vi "TL forebrain THINK.vi"(7 "MDF":T1(array[cluster]), 8 "error in":errorcluster, 9 "Run?":bool=TRUE, 10 "MDF index":i32, 11 "GPS":cluster{"X pos":i32, "Y pos":i32, "Heading":dbl}={"X pos"=250, "Y pos"=250, "Heading"=0.0}) -> (0 "error out":errorcluster, 1 "local Steering\nangle":dbl, 2 "MDF Index out":i32, 3 "Behaviors out":T2, 5 "MDF Out":T1(array[cluster]), 6 "Complete?":bool=TRUE)   [LabVIEW 2014]
panel:
  out "At Waypoint?":bool
  out "Forebrain Command":T3
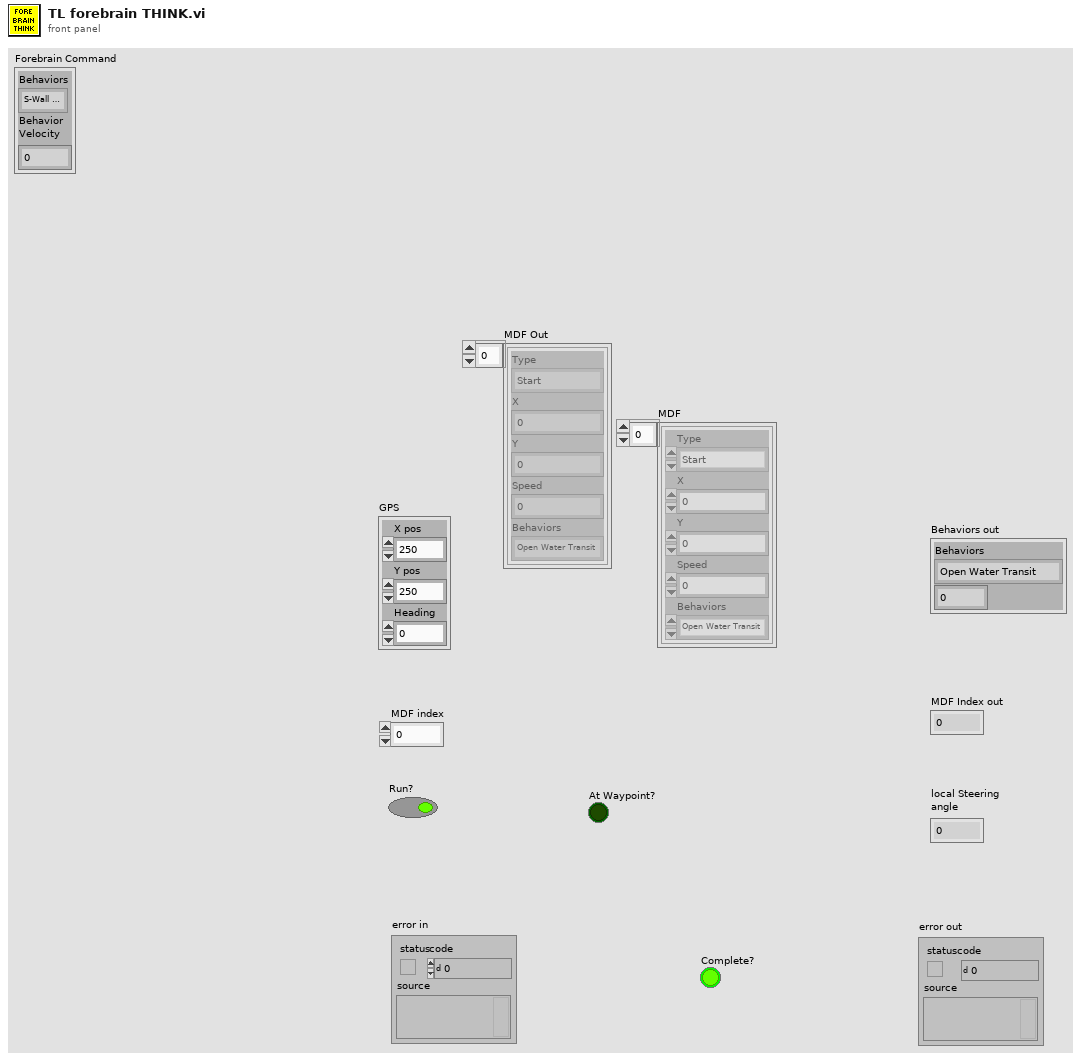
[diagram p1: front panel]
types:
  T1 = cluster{"Type":enum16{"Start", "Buoy Circling", "Waypoint", "End"}, "X":i32, "Y":i32, "Speed":i32, "Behaviors":enum16{"Open Water Transit", "P-Wall Follow", "S-Wall Follow", "Get Unstuck"}}[]
  T2 = cluster{"Behaviors":enum16{"Open Water Transit", "P-Wall Follow", "S-Wall Follow", "Get Unstuck"}, dbl}
  T3 = cluster{"Behaviors":enum16{"S-Wall Follow", "P-Wall Follow", "Open Water Transit", "Get Unstuck"}, "Behavior\nVelocity":dbl}
  T4 = enum16{"Open Water Transit", "P-Wall Follow", "S-Wall Follow", "Get Unstuck"}
  T5 = cluster{"Type":enum16{"Start", "Buoy Circling", "Waypoint", "End"}, "X":i32, "Y":i32, "Speed":i32, "Behaviors":enum16{"Open Water Transit", "P-Wall Follow", "S-Wall Follow", "Get Unstuck"}}
  T6 = enum16{"Start", "Buoy Circling", "Waypoint", "End"}
  T7 = cluster{"Pos. X":i32, "Pos. Y":i32, "Radius":i32, "Core Area":i32}[]
  T8 = cluster{"Pos. X":i32, "Pos. Y":i32, "Radius":i32, "Core Area":i32}
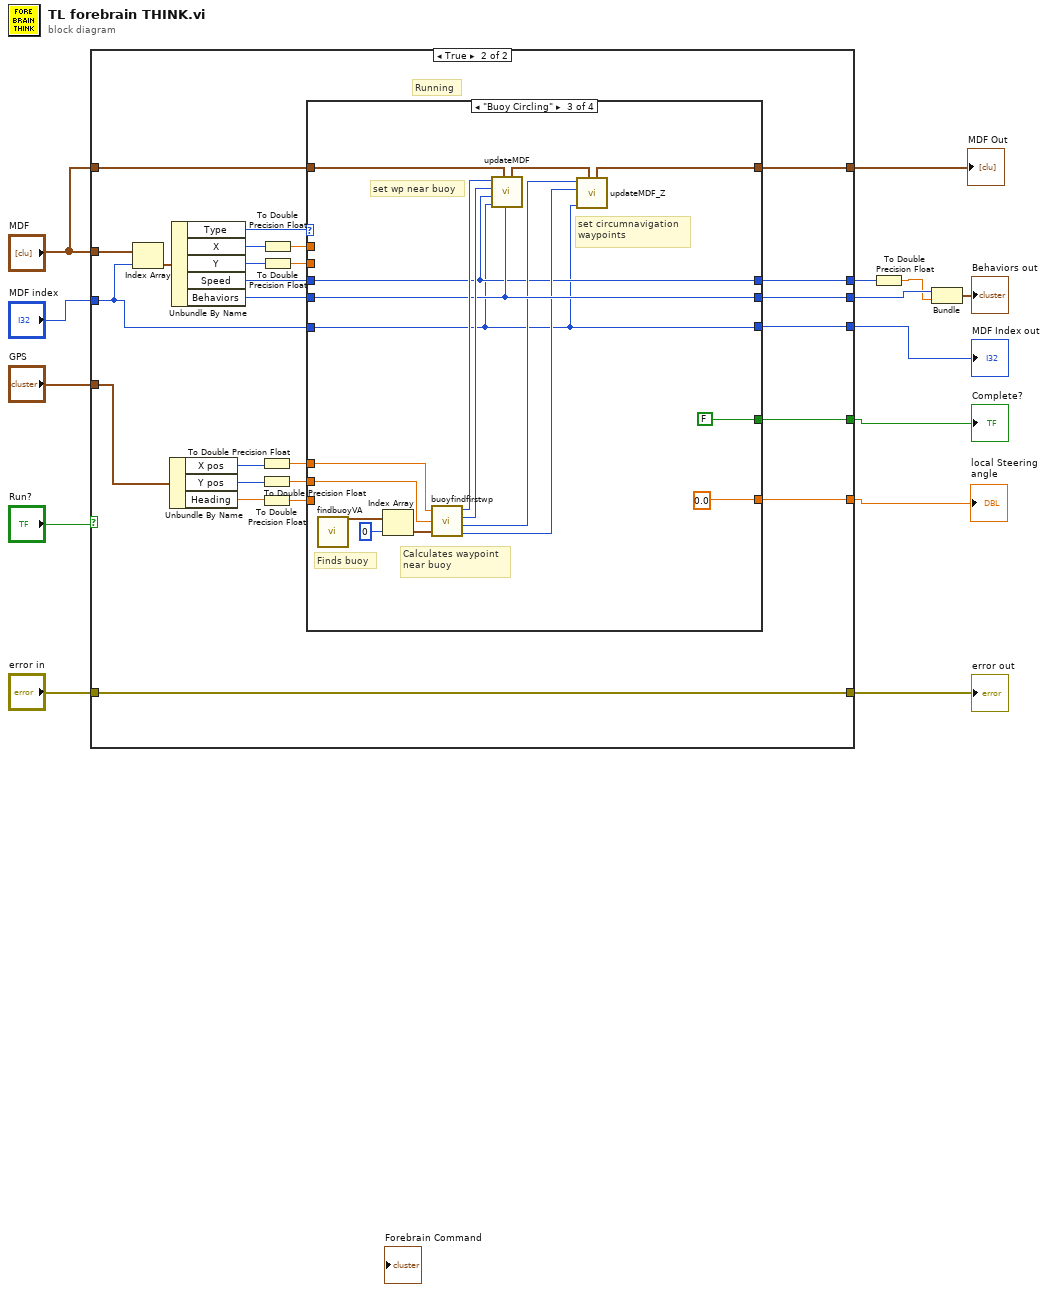
[diagram p0: block diagram]
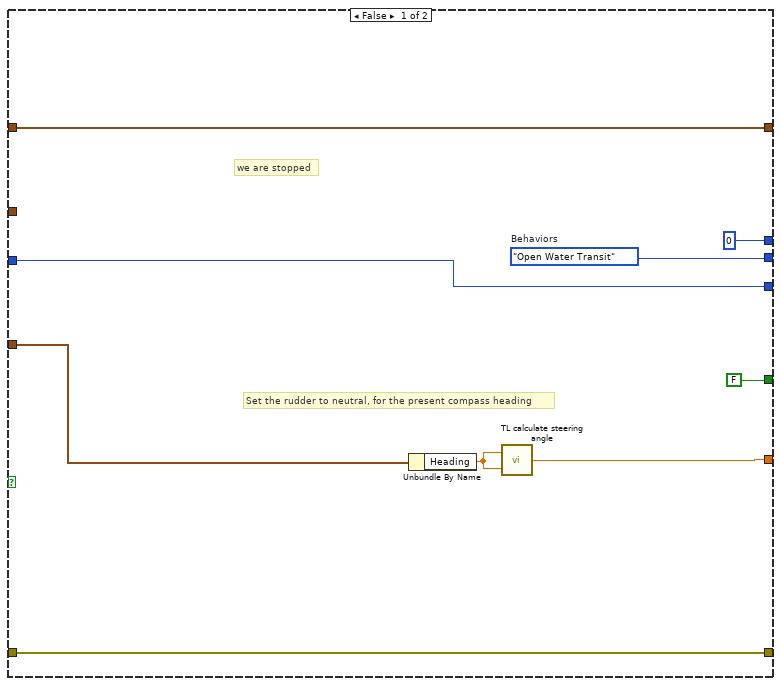
[diagram p2: hidden frame]
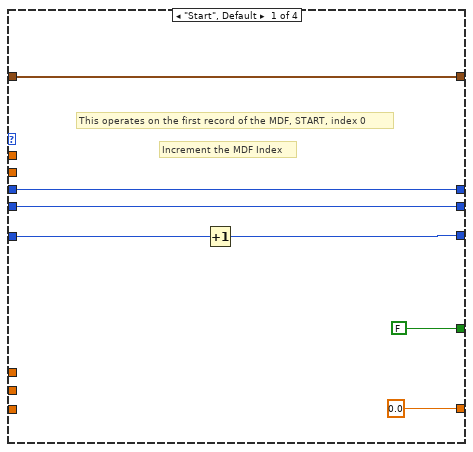
[diagram p3: hidden frame]
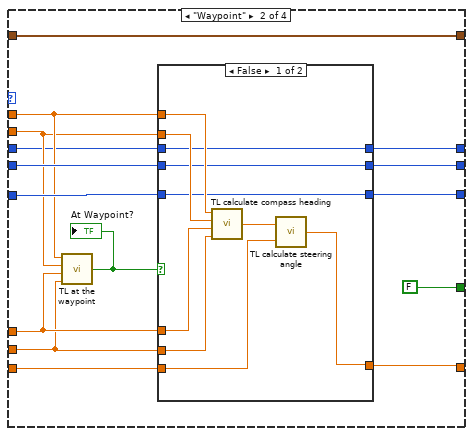
[diagram p4: hidden frame]
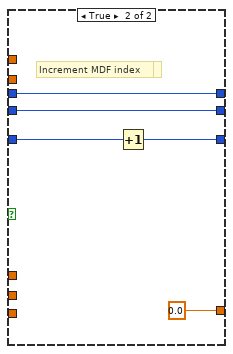
[diagram p5: hidden frame]
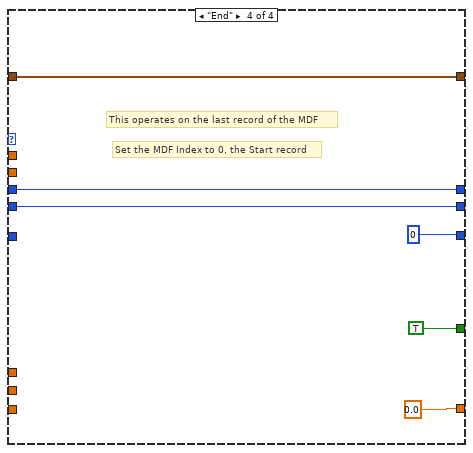
[diagram p6: hidden frame]
diagram:
  n1 = case shown="True" "Run?" {
    tunnel: "MDF" -> [_ w48]
    tunnel: "MDF index" -> [w19 w33]
    tunnel: "error in" -> [w23 w45]
    tunnel: [w23 w45] -> w12
    tunnel: "GPS" -> [w22 w44]
    tunnel: [w19 w31] -> w9
    tunnel: [w20 w30] -> w8
    tunnel: [0 w28] -> w7
    tunnel: [w17 w27] -> w6
    tunnel: [FALSE w26] -> w3
    tunnel: [w15 w25] -> w1
    tunnel: "MDF" -> [w15 w24]
    frame False {
      w17 = T4."Open Water Transit"  # Behaviors
      # "Set the rudder to neutral, for the present compass heading"
      # "we are stopped"
      n2 = Unbundle By Name(w22) -> ("Heading"=w21:dbl)
      n3 = call "TL calculate steering angle.vi"("Compass\nheading"=w21, "New heading"=w21) -> ("Local Steering Angle"=w20:dbl)
    }
    frame True {
      # "Running"
      n4 = Index Array(array=w48, index=w33) -> (element=w47:T5)
      n5 = Unbundle By Name(w44) -> ("X pos"=w41:i32, "Y pos"=w39:i32, "Heading"=w40:dbl)
      n6 = Unbundle By Name(w47) -> ("Type"=w46:T6, "X"=w42:i32, "Y"=w43:i32, "Speed"=w29:i32, "Behaviors"=w32:T4)
      n7 = To Double Precision Float(number=w41) -> (double precision float=w36:dbl)
      n8 = To Double Precision Float(number=w39) -> (double precision float=w35:dbl)
      n9 = To Double Precision Float(number=w40) -> (double precision float=w34:dbl)
      n10 = To Double Precision Float(number=w42) -> (double precision float=w38:dbl)
      n11 = To Double Precision Float(number=w43) -> (double precision float=w37:dbl)
      n12 = case shown="\"Buoy Circling\"" w46 {
        tunnel: w38 -> [_ w61 _ _]
        tunnel: w37 -> [_ w60 _ _]
        tunnel: w36 -> [_ w64 w97 _]
        tunnel: w35 -> [_ w63 w98 _]
        tunnel: w34 -> [_ w62 _ _]
        tunnel: w33 -> [w53 w67 w87 _]
        tunnel: [w52 w66 w87 0] -> w31
        tunnel: w32 -> [w55 w69 w92 w108]
        tunnel: [w55 w68 w92 w108] -> w27
        tunnel: [0.0 w65 0.0 0.0] -> w30
        tunnel: w29 -> [w51 w59 w89 w105]
        tunnel: [w51 w58 w89 w105] -> w28
        tunnel: [FALSE FALSE FALSE TRUE] -> w26
        tunnel: [w49 w56 w86 w103] -> w25
        tunnel: w24 -> [w49 w56 w100 w103]
        frame "Start", Default {
          # "Increment the MDF Index"
          # "This operates on the first record of the MDF, START, index 0"
          n13 = Increment(x=w53) -> (x+1=w52:i32)
        }
        frame "Waypoint" {
          n14 = call "TL at the waypoint.vi"("Y location"=w63, "X location"=w64, "Yof waypoint"=w60, "X of waypoint"=w61) -> ("At Waypoint?"=w70:bool)
          "At Waypoint?" <- w70
          n15 = case shown="False" w70 {
            tunnel: w69 -> [w72 w85]
            tunnel: [w72 w85] -> w68
            tunnel: w67 -> [w73 w84]
            tunnel: [w73 w83] -> w66
            tunnel: [w74 0.0] -> w65
            tunnel: w64 -> [w78 _]
            tunnel: w63 -> [w77 _]
            tunnel: w62 -> [w75 _]
            tunnel: w61 -> [w80 _]
            tunnel: w60 -> [w79 _]
            tunnel: w59 -> [w71 w81]
            tunnel: [w71 w81] -> w58
            frame False {
              n16 = call "TL calculate compass heading.vi"("Y Location"=w77, "X Location"=w78, "Waypoint Y"=w79, "Waypoint X"=w80) -> ("Heading"=w76:dbl)
              n17 = call "TL calculate steering angle.vi"("Compass\nheading"=w75, "New heading"=w76) -> ("Local Steering Angle"=w74:dbl)
            }
            frame True {
              # "We are at the waypoint"
              # "Increment MDF index"
              n18 = Increment(x=w84) -> (x+1=w83:i32)
            }
          }
        }
        frame "Buoy Circling" {
          # "Finds buoy"
          # "set circumnavigation\nwaypoints"
          # "set wp near buoy"
          # "Calculates waypoint\nnear buoy"
          n19 = call "findbuoyVA.vi"() -> ("Circles Data (Circle Detection 1)"=w102:T7)  [unwired: 26 in, 1 out]
          n20 = Index Array(array=w102, index=0) -> (element=w99:T8)
          n21 = call "buoyfindfirstwp.vi"("X of boat"=w97, "Y of boat"=w98, "Buoy Location Input"=w99) -> ("X of new waypoint"=w96:i32, "Y of new waypoint"=w95:i32, "X of Buoy"=w91:i32, "Y of Buoy"=w90:i32)
          n22 = call "updateMDF.vi"("Behaviors"=w92, "MDF"=w100, "MDF Index to Change"=w87, "Speed"=w89, "Y new wp"=w95, "X new wp"=w96) -> ("New MDF"=w88:T1)  [unwired: 5 in]
          n23 = call "updateMDF_Z.vi"("MDF"=w88, "index"=w87, "buoy Y"=w90, "buoy X"=w91) -> ("MDF out"=w86:T1)  [unwired: 5 in, 2 out]
        }
        frame "End" {
          # "Set the MDF Index to 0, the Start record"
          # "This operates on the last record of the MDF"
        }
      }
    }
  }
  "error out" <- w12
  "local Steering\nangle" <- w8
  "MDF Index out" <- w9
  "Complete?" <- w3
  "MDF Out" <- w1
  n24 = To Double Precision Float(number=w7) -> (double precision float=w5:dbl)
  n25 = Bundle("Behaviors"=w6, w5) -> (→"Behaviors out":T2)  [unwired: 1 in]
